vi "Procesamiento_d_imagen.vi"() -> ()   [LabVIEW 2021]
uses:
  <vilib>/picture/picture.llb/imagedata.ctl
panel:
  in  "Slide":cluster{u8, u8, u8}(slide)={0, 22, 88} scale=0.0..255.0
  out "new picture 2":picture
  out "image data":T1
  in  "Path":path
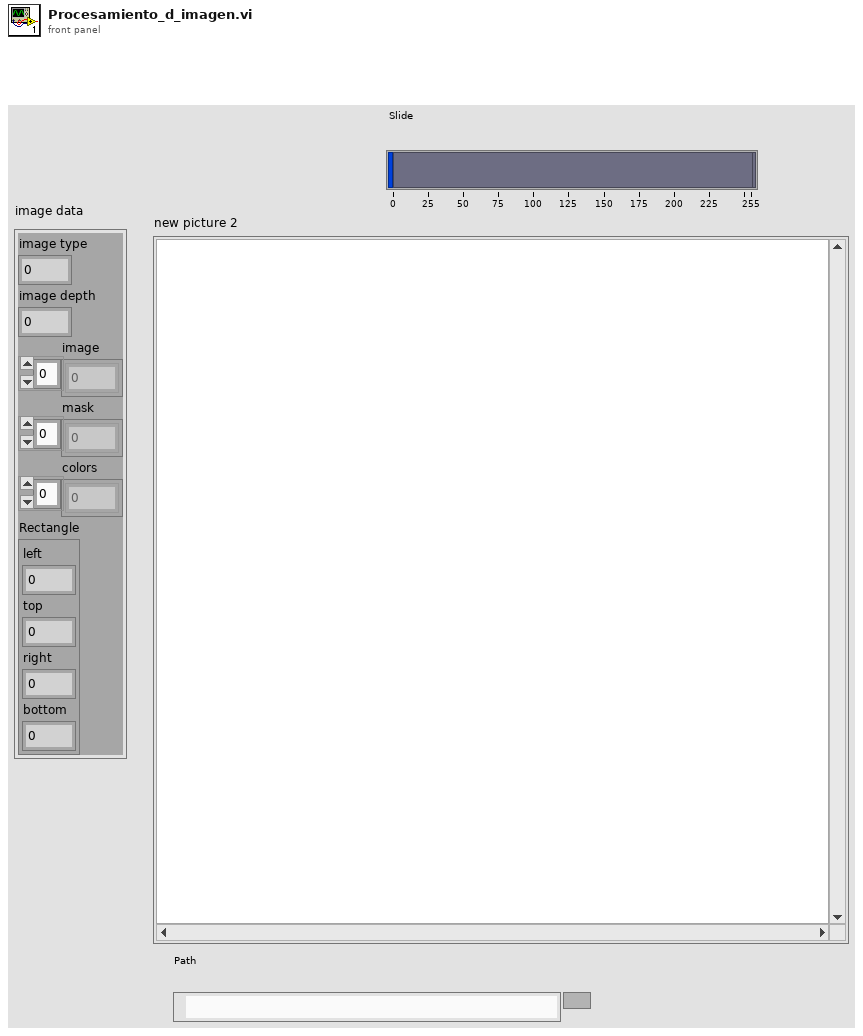
[diagram p1: front panel]
types:
  T1 = typedef "imagedata.ctl" = cluster{"image type":i32, "image depth":i32, "image":u8[], "mask":u8[], "colors":u32[], "Rectangle":cluster{"left":i16, "top":i16, "right":i16, "bottom":i16}}
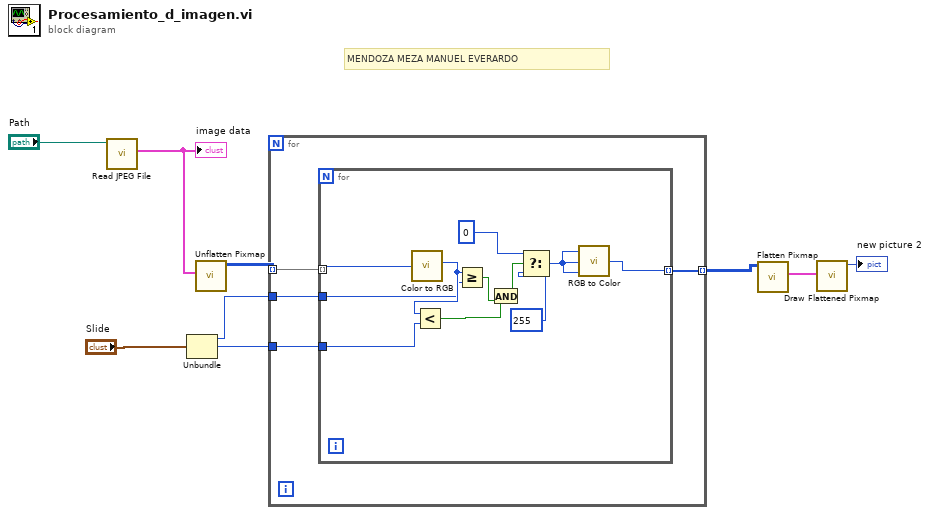
[diagram p0: block diagram]
diagram:
  # "MENDOZA MEZA MANUEL EVERARDO"
  n1 = call <vilib>:"Read JPEG File.vi"("path to JPEG file"="Path") -> ("image data"=w8:T1)  [unwired: 8 in, 2 out]
  "image data" <- w8
  n2 = Unbundle("Slide") -> (w2:u8, w1:u8)  [unwired: 1 out]
  n3 = call <vilib>:"Unflatten Pixmap.vi"("image data"=w8) -> ("24-bit pixmap"=w7:u32[][])  [unwired: 4 in, 6 out]
  n4 = for {
    tunnel: w7 -> [w13] mode=indexing
    tunnel: [w12] -> w6 mode=indexing
    tunnel: w2 -> [w11]
    tunnel: w1 -> [w10]
    n5 = for {
      tunnel: w13 -> [w24] mode=indexing
      tunnel: [w23] -> w12 mode=indexing
      tunnel: w11 -> [w15]
      tunnel: w10 -> [w14]
      n6 = call <vilib>:"Color to RGB.vi"("Color"=w24) -> ("R"=w19:u8)  [unwired: 3 out]
      n7 = Less?(x=w19, y=w14) -> (x < y?=w18:bool)
      n8 = Greater Or Equal?(x=w19, y=w15) -> (x >= y?=w17:bool)
      n9 = And(x=w18, y=w17) -> (x .and. y?=w16:bool)
      n10 = Select(t=0, s=w16, f=255) -> (s? t:f=w20:i32)
      n11 = call <vilib>:"RGB to Color.vi"("B"=w20, "G"=w20, "R"=w20) -> ("Color"=w23:u32)
    }
  }
  n12 = call <vilib>:"Flatten Pixmap.vi"("24-bit pixmap"=w6) -> ("image data"=w5:T1)  [unwired: 10 in]
  n13 = call <vilib>:"Draw Flattened Pixmap.vi"("image data"=w5) -> ("new picture"=→"new picture 2":picture)  [unwired: 8 in]
